vi "mgcVI.vi"() -> ()   [LabVIEW 2018]
uses:
  <vilib>/Instr/_visa.llb/VISA Configure Serial Port (Instr).vi
panel:
  in  "stop 2":bool
  out "read buffer 2":string
  in  "VISA resource name":refnum<visa-resource-name>
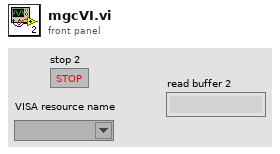
[diagram p1: front panel]
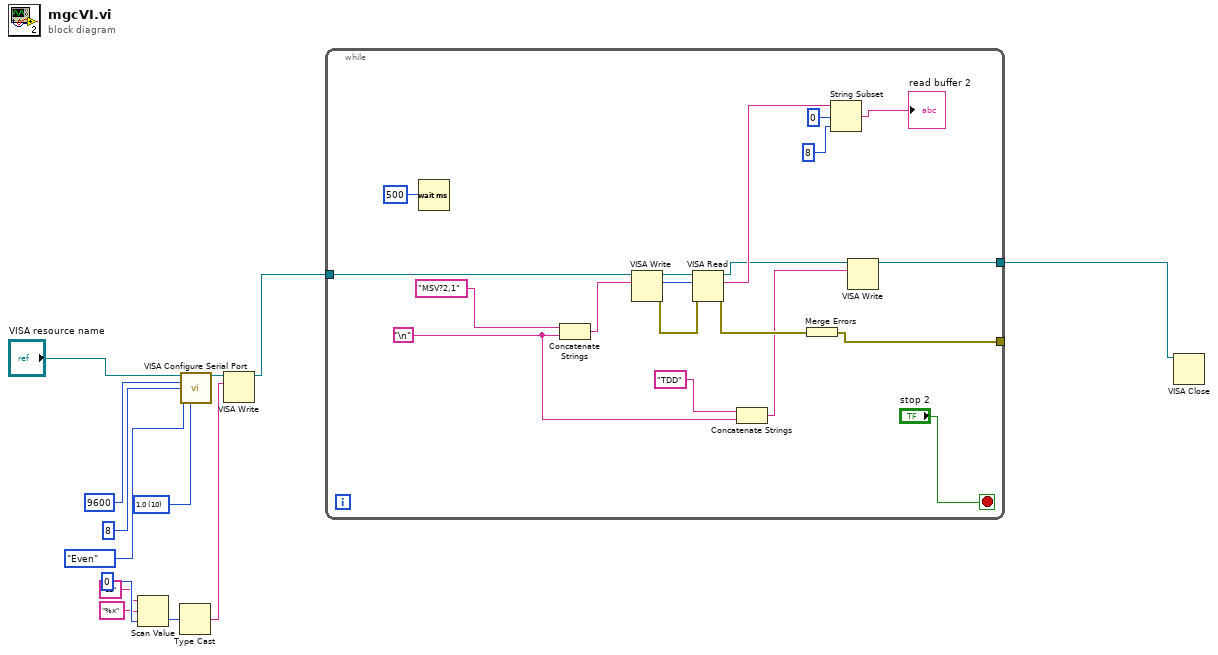
[diagram p0: block diagram]
diagram:
  w9 = u16 10 items=["1.0"=10, "1.5"=15, "2.0"=20] ("stop bits (10: 1 bit)")
  n1 = Scan Value(string="12", format string="%x", default (0 dbl)=0) -> (value=w3:i32)  [unwired: 1 out]
  n2 = Type Cast(x=w3) -> (*(type *) &x=w4:string)  [unwired: 1 in]
  n3 = call-poly "VISA Configure Serial Port"("VISA resource name"="VISA resource name", "baud rate (9600)"=u32 9600, "data bits (8)"=u16 8, "parity (0:none)"=enum16{"None", "Odd", "Even", "Mark", "Space"}."Even", "stop bits (10: 1 bit)"=w9) -> ("VISA resource name out"=w5:refnum<visa-resource-name>)  [unwired: 9 in, 1 out]
  n4 = VISA Write(VISA resource name=w5, write buffer=w4) -> (VISA resource name out=w2:refnum<visa-resource-name>)  [unwired: 1 in, 2 out]
  n5 = while {
    tunnel: w2 -> [w20]
    tunnel: [w19] -> _
    tunnel: [w17] -> w1
    stop <- "stop 2" stop-if-true
    w15 = "\n"
    n6 = Wait (ms)(milliseconds to wait=u32 500) -> ()  [unwired: 1 out]
    n7 = Concatenate Strings("MSV?2,1" ("write buffer"), w15) -> (w26:string)
    n8 = VISA Write(VISA resource name=w20, write buffer=w26) -> (VISA resource name out=w27:refnum<visa-resource-name>, return count=w31:u32, error out=w32:errorcluster)  [unwired: 1 in]
    n9 = VISA Read(VISA resource name=w27, byte count=w31, error in (no error)=w32) -> (VISA resource name out=w18:refnum<visa-resource-name>, read buffer=w28:string, error out=w30:errorcluster)  [unwired: 1 out]
    n10 = Concatenate Strings("TDD" ("string"), w15) -> (w14:string)
    n11 = Merge Errors(w30) -> (w19:errorcluster)
    n12 = String Subset(string=w28, offset (0)=0, length (rest)=8 ("length (rest)")) -> (substring=→"read buffer 2":string)
    n13 = VISA Write(VISA resource name=w18, write buffer=w14) -> (VISA resource name out=w17:refnum<visa-resource-name>)  [unwired: 1 in, 2 out]
  }
  n14 = VISA Close(VISA resource name=w1) -> ()  [unwired: 1 in, 1 out]
